vi "SA Cond - Time Varying Metrics.vi"(0 "wForm IN":waveform(dbl)[](array[waveform]), 5 "error in (no error)":errorcluster, 6 "Nb Signals":i32, 7 "Trend Type":T1(ring) caption="Type", 8 "Anotate Signal Name":bool=TRUE, 9 "Step (ms)":dbl=10.0 min=1.0 max=10000.0 step=1.0, 11 "Length (ms)":dbl=125.0) -> (14 "wForm OUT":waveform(dbl)[](array[waveform]), 19 "error out":errorcluster)   [LabVIEW 2022 SP3, in "GSwFormDSP.lvclass"]
uses:
  GSwFormDSP.lvclass
  functions/Attribute List.ctl
  functions/Attribute Options.ctl
  <vilib>/Analysis/NI_AALBase.lvlib
  <vilib>/Analysis/NI_AALPro.lvlib
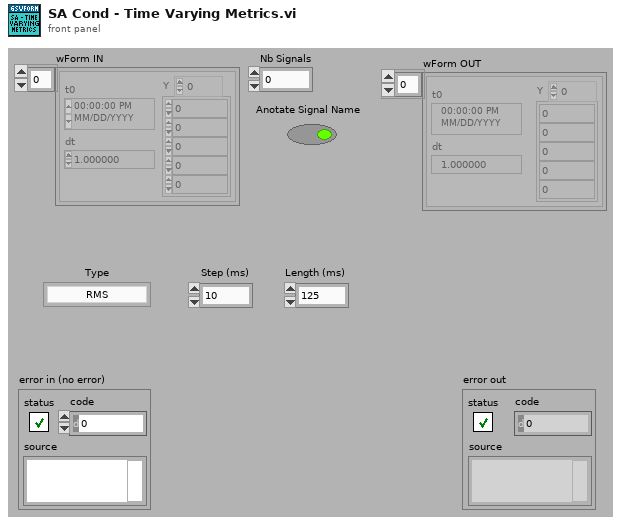
[diagram p1: front panel]
types:
  T1 = enum16{"RMS", "Absolute Peak", "Range", "Standard Deviation", "Variance", "Skewness", "Kurtosis"}
  T2 = typedef "GSwFormDSP.lvclass/Attribute Options.ctl" = enum16{"Append to Attribute using \"( )\"", "Replace Attribute Value"}
  T3 = typedef "GSwFormDSP.lvclass/Attribute List.ctl" = string
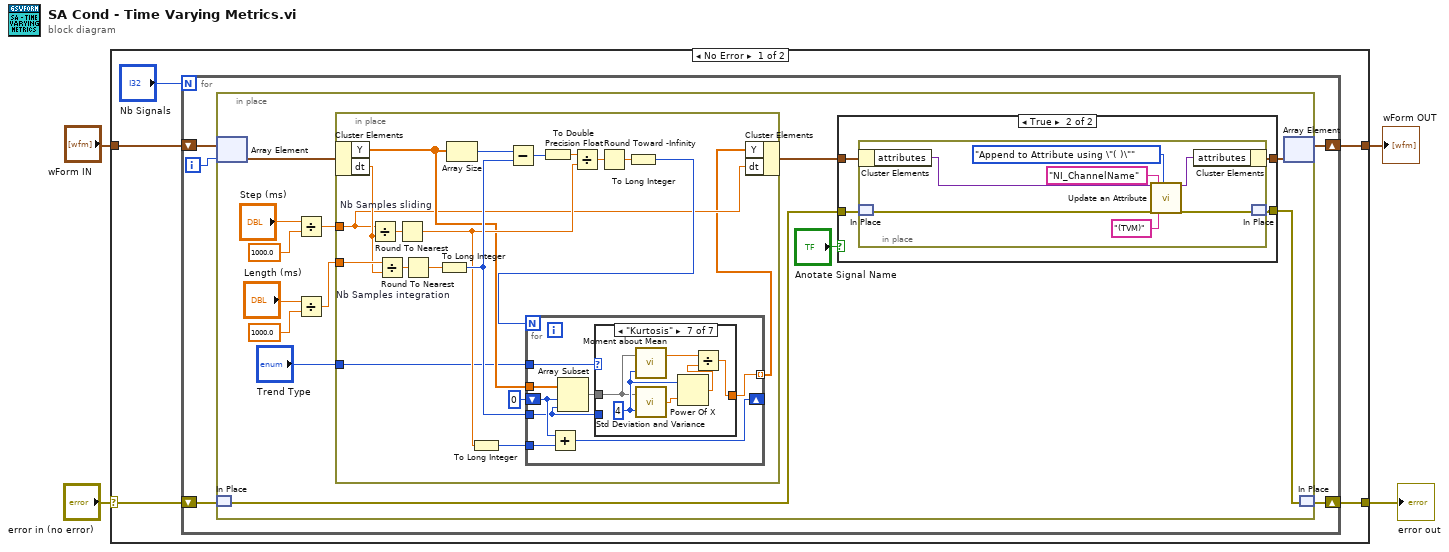
[diagram p0: block diagram]
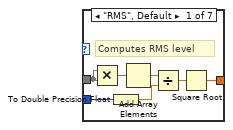
[diagram p2: hidden frame]
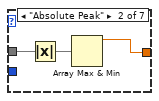
[diagram p3: hidden frame]
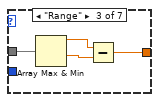
[diagram p4: hidden frame]
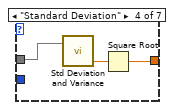
[diagram p5: hidden frame]
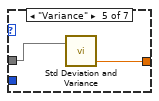
[diagram p6: hidden frame]
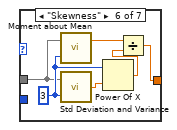
[diagram p7: hidden frame]
diagram:
  n1 = case shown="No Error" "error in (no error)" {
    selector: "error in (no error)" -> [w8 w100]
    tunnel: [w6 w100] -> w3
    tunnel: "wForm IN" -> [w9 w99]
    tunnel: [w7 w99] -> w1
    frame No Error {
      n2 = for {
        N: "Nb Signals" -> [_]
        shift-right: [w13] -> w7
        shift-left: w9 -> [w12]
        shift-right: [w10] -> w6
        shift-left: w8 -> [w11]
        i -> [w14]
        n3 = in-place {
          n4 = in-place-array #1(w12, w14) -> (w24:waveform(dbl))
          n5 = in-place-match #2(w11) -> (w15:errorcluster)
          n6 = Divide(x="Step (ms)", y=1000.0 ("x")) -> (x/y=w18:dbl)
          n7 = Divide(x="Length (ms)", y=1000.0 ("x")) -> (x/y=w17:dbl)
          n8 = in-place {
            in-place-border: w18 -> [w31]
            in-place-border: w17 -> [w38]
            in-place-border: "Trend Type" -> [w28]
            n9 = in-place-cluster #3(w24) -> ("Y"=w33:dbl[], "dt"=w32:dbl)
            n10 = Divide "Nb Samples sliding"(x=w31, y=w32) -> (x/y=w39:dbl)
            n11 = Divide "Nb Samples integration"(x=w38, y=w32) -> (x/y=w40:dbl)
            n12 = Round To Nearest(number=w39) -> (nearest integer value=w35:dbl)
            n13 = Round To Nearest(number=w40) -> (nearest integer value=w41:dbl)
            n14 = To Long Integer(number=w41) -> (32bit integer=w36:i32)
            n15 = Array Size(array=w33) -> (size(s)=w42:i32)
            n16 = To Long Integer(number=w35) -> (32bit integer=w34:i32)
            n17 = Subtract(x=w42, y=w36) -> (x-y=w46:i32)
            n18 = To Double Precision Float(number=w46) -> (double precision float=w43:dbl)
            n19 = Divide(x=w43, y=w35) -> (x/y=w44:dbl)
            n20 = Round Toward -Infinity(1:w44) -> (0:w45:dbl)
            n21 = To Long Integer(number=w45) -> (32bit integer=w37:i32)
            n22 = for {
              N: w37 -> [_]
              shift-right: [w51] -> _
              shift-left: 0 -> [w53]
              tunnel: w36 -> [w49]
              tunnel: w33 -> [w54]
              tunnel: w34 -> [w52]
              tunnel: [w50] -> w30 mode=indexing
              tunnel: w28 -> [w47]
              n23 = Add(x=w53, y=w52) -> (x+y=w51:i32)
              n24 = Array Subset(array=w54, index=w53, length=w49) -> (w48:dbl[])
              n25 = case shown="\"Kurtosis\"" w47 {
                tunnel: [w61 w62 w65 w69 w72 w74 w80] -> w50
                tunnel: w49 -> [w60 _ _ _ _ _ _]
                tunnel: w48 -> [w59 w64 w68 w70 w73 w76 w82]
                frame "RMS", Default {
                  # "Computes RMS level"
                  n26 = Multiply(x=w59, y=w59) -> (x*y=w55:dbl[])
                  n27 = To Double Precision Float(number=w60) -> (double precision float=w57:dbl)
                  n28 = Add Array Elements(numeric array=w55) -> (sum=w56:dbl)
                  n29 = Divide(x=w56, y=w57) -> (x/y=w58:dbl)
                  n30 = Square Root(x=w58) -> (sqrt(x)=w61:dbl)
                }
                frame "Absolute Peak" {
                  n31 = Absolute Value(x=w64) -> (abs(x)=w63:dbl[])
                  n32 = Array Max & Min(array=w63) -> (max value=w62:dbl)  [unwired: 3 out]
                }
                frame "Range" {
                  n33 = Array Max & Min(array=w68) -> (max value=w67:dbl, min value=w66:dbl)  [unwired: 2 out]
                  n34 = Subtract(x=w67, y=w66) -> (x-y=w65:dbl)
                }
                frame "Standard Deviation" {
                  n35 = call <vilib>:"Std Deviation and Variance.vi"("X"=w70) -> ("variance"=w71:dbl)  [unwired: 1 in, 2 out]
                  n36 = Square Root(x=w71) -> (sqrt(x)=w69:dbl)
                }
                frame "Variance" {
                  n37 = call <vilib>:"Std Deviation and Variance.vi"("X"=w73) -> ("variance"=w72:dbl)  [unwired: 1 in, 2 out]
                }
                frame "Skewness" {
                  w79 = 3
                  n38 = call <vilib>:"Moment about Mean.vi"("order"=w79, "X"=w76) -> ("moment"=w77:dbl)  [unwired: 1 out]
                  n39 = call <vilib>:"Std Deviation and Variance.vi"("X"=w76, "Weighting (Sample)"=w79) -> ("standard deviation"=w78:dbl)  [unwired: 2 out]
                  n40 = Power Of X(1:w78, 2:w79) -> (0:w75:dbl)
                  n41 = Divide(x=w77, y=w75) -> (x/y=w74:dbl)
                }
                frame "Kurtosis" {
                  w85 = 4
                  n42 = call <vilib>:"Moment about Mean.vi"("order"=w85, "X"=w82) -> ("moment"=w83:dbl)  [unwired: 1 out]
                  n43 = call <vilib>:"Std Deviation and Variance.vi"("X"=w82, "Weighting (Sample)"=w85) -> ("standard deviation"=w84:dbl)  [unwired: 2 out]
                  n44 = Power Of X(1:w84, 2:w85) -> (0:w81:dbl)
                  n45 = Divide(x=w83, y=w81) -> (x/y=w80:dbl)
                }
              }
            }
            n46 = in-place-cluster #3("Y"=w30, "dt"=w31) -> (w23:waveform(dbl))
          }
          n47 = case shown="True" "Anotate Signal Name" {
            tunnel: [w86 w91] -> w26
            tunnel: [w87 w90] -> w25
            tunnel: w23 -> [w86 w89]
            tunnel: w15 -> [w87 w88]
            frame False {
            }
            frame True {
              n48 = in-place {
                n49 = in-place-cluster #4(w89) -> ("attributes"=w98:variant)
                n50 = in-place-match #5(w88) -> (w92:errorcluster)
                n51 = call "Update an Attribute.vi"("attributes in"=w98, "error in (no error)"=w92, "Attribute List"=T3 "NI_ChannelName", "Attribute Value"="(TVM)" ("string"), "Attribute Option"=Attribute_Options."Append to Attribute using \"( )\"") -> ("attributes out"=w97:variant, "error out"=w96:errorcluster)  [unwired: 13 in]
                n52 = in-place-cluster #4("attributes"=w97) -> (w91:waveform(dbl))
                n53 = in-place-match #5(w96) -> (w90:errorcluster)
              }
            }
          }
          n54 = in-place-array #1(w26) -> (w13:waveform(dbl)[])  [unwired: 1 out]
          n55 = in-place-match #2(w25) -> (w10:errorcluster)
        }
      }
    }
    frame Error {
    }
  }
  "error out" <- w3
  "wForm OUT" <- w1
